vi "get-data.vi"(3 "error in (no error)":errorcluster, 4 "andor-get-data-cluster":T2={"detector"=0, "HBinning"=1, "readout mode"=0} {"readout mode" items=["Full Vertical Binning", "Image", "Vertical Binning"]; "HBinning" items=["1x"=1, "2x"=2, "4x"=4, "8x"=8, "16x"=16]; "detector" items=["Newton", "iDus", "Clara", "Xeva"]}, 5 "xeva-camref-in":T3) -> (0 "error out":errorcluster, 1 "raw-data":i32[](array[numeric]), 2 "xeva-camref-out":T3)   [LabVIEW 2015]
uses:
  <vilib>/Xenics Infrared Solutions/Xeneth LabVIEW API/VIs/Controls/Camara.ctl
  <userlib>/atmcd32d.llb/Error Code Enum typedef.ctl
  <vilib>/Xenics Infrared Solutions/Xeneth LabVIEW API/Xeneth.lvlib
panel:
  out "Get Data Status":T1=enum."DRV_SUCCESS"
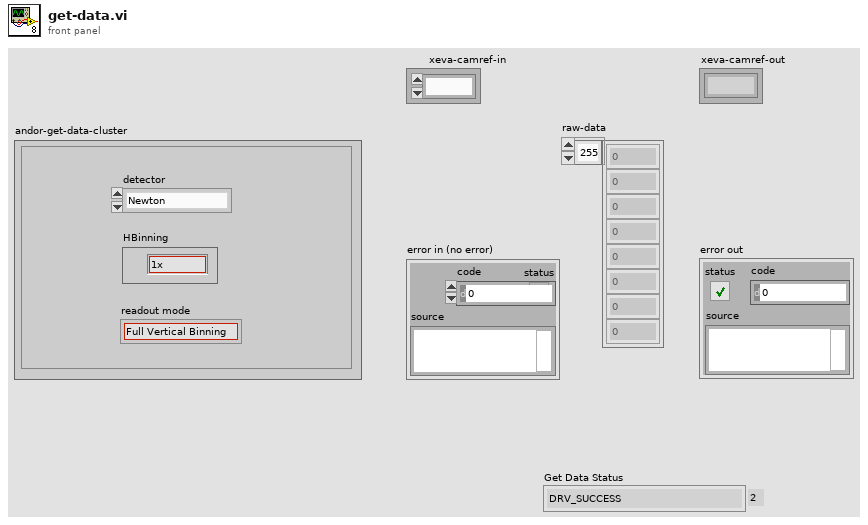
[diagram p1: front panel]
types:
  T1 = typedef "Error Code Enum typedef.ctl" = enum32{"N/A (0)", "DRV_ERROR_CODES", "DRV_SUCCESS", "DRV_VXDNOTINSTALLED", "DRV_ERROR_SCAN", "DRV_ERROR_CHECK_SUM", "DRV_ERROR_FILELOAD", "DRV_UNKNOWN_FUNC", "DRV_ERROR_VXD_INIT", "DRV_ERROR_ADDRESS", "DRV_ERROR_PAGELOCK", "DRV_ERROR_PAGEUNLOCK", "DRV_ERROR_BOARDTEST", "DRV_ERROR_ACK", "DRV_ERROR_UP_FIFO", "DRV_ERROR_PATTERN", "N/A (16)", "DRV_ACQUISITION_ERRORS", "DRV_ACQ_BUFFER", "DRV_ACQ_DOWNFIFO_FULL", "DRV_PROC_UNKONWN_INSTRUCTION", "DRV_ILLEGAL_OP_CODE", "DRV_KINETIC_TIME_NOT_MET", "DRV_ACCUM_TIME_NOT_MET", "DRV_NO_NEW_DATA", "N/A (25)", "DRV_SPOOLERROR", "N/A (27)", "N/A (28)", "N/A (29)", "N/A (30)", "N/A (31)", "N/A (32)", "DRV_TEMPERATURE_CODES", "DRV_TEMPERATURE_OFF", "DRV_TEMPERATURE_NOT_STABILIZED", "DRV_TEMPERATURE_STABILIZED", "DRV_TEMPERATURE_NOT_REACHED", "DRV_TEMPERATURE_OUT_RANGE", "DRV_TEMPERATURE_NOT_SUPPORTED", "DRV_TEMPERATURE_DRIFT", "N/A (41)", "N/A (42)", "N/A (43)", "N/A (44)", "N/A (45)", "N/A (46)", "N/A (47)", "N/A (48)", "DRV_GENERAL_ERRORS", "DRV_INVALID_AUX", "DRV_COF_NOTLOADED", "DRV_FPGAPROG", "DRV_FLEXERROR", "DRV_GPIBERROR", "N/A (55)", "N/A (56)", "N/A (57)", "N/A (58)", "N/A (59)", "N/A (60)", "N/A (61)", "N/A (62)", "N/A (63)", "DRV_DATATYPE", "DRV_DRIVER_ERRORS", "DRV_P1INVALID", "DRV_P2INVALID", "DRV_P3INVALID", "DRV_P4INVALID", "DRV_INIERROR", "DRV_COFERROR", "DRV_ACQUIRING", "DRV_IDLE", "DRV_TEMPCYCLE", "DRV_NOT_INITIALIZED", "DRV_P5INVALID", "DRV_P6INVALID", "DRV_INVALID_MODE", "DRV_INVALID_FILTER", "DRV_I2CERRORS", "DRV_I2CDEVNOTFOUND", "DRV_I2CTIMEOUT", "DRV_P7INVALID", "N/A (84)", "N/A (85)", "N/A (86)", "N/A (87)", "N/A (88)", "N/A (89)", "DRV_IOCERROR", "DRV_VRMVERSIONERROR"}
  T2 = cluster{"detector":u16, "HBinning":u16, "readout mode":u16}
  T3 = typedef "Xeneth.lvlib/Camara.ctl" = refnum<k1>
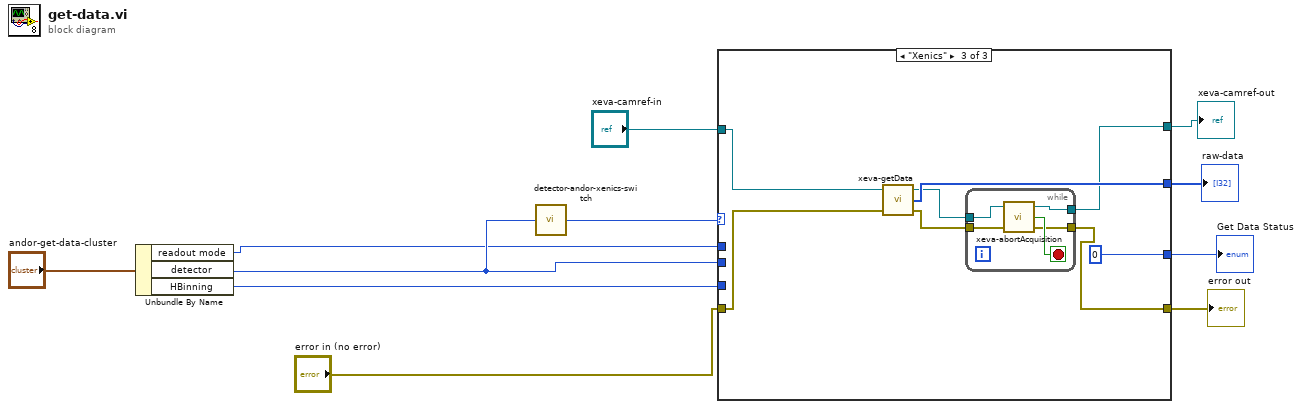
[diagram p0: block diagram]
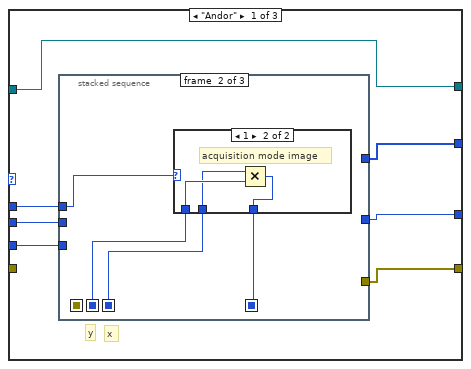
[diagram p2: hidden frame]
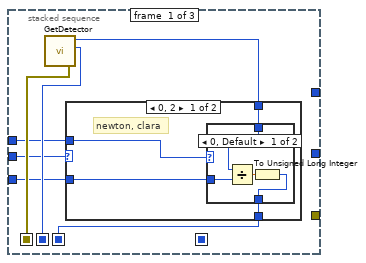
[diagram p3: hidden frame]
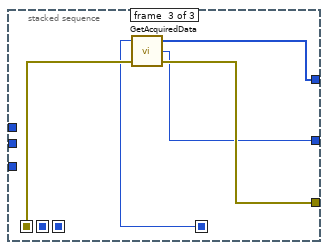
[diagram p7: hidden frame]
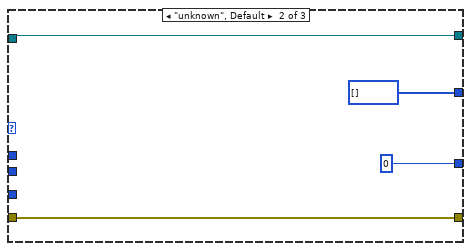
[diagram p8: hidden frame]
diagram:
  n1 = Unbundle By Name("andor-get-data-cluster") -> ("readout mode"=w5:u16, "detector"=w6:u16, "HBinning"=w4:u16)
  n2 = call "detector-andor-xenics-switch.vi"("Detector"=w6) -> ("Manufacturer"=w7:enum16{"Andor", "Xenics", "unknown"})
  n3 = case shown="\"Xenics\"" w7 {
    tunnel: [w13 w52 w53] -> w11
    tunnel: "error in (no error)" -> [_ w52 w59]
    tunnel: "xeva-camref-in" -> [w18 w51 w58]
    tunnel: [w18 w51 w55] -> w8
    tunnel: w5 -> [w17 _ _]
    tunnel: w4 -> [w16 _ _]
    tunnel: w6 -> [w15 _ _]
    tunnel: [w14 u32 0 ("DLL error code") u32 0 ("DLL error code")] -> w2
    tunnel: [w12 i32[] [] ("array") w57] -> w1
    frame "Andor" {
      # "x"
      # "y"
      n4 = stacked-sequence {
        seq-local: [w24 _ _] -> [_ w39 _]
        seq-local: [w23 _ _] -> [_ w38 _]
        seq-local: [_ w37 _] -> [_ _ w46]
        seq-local: [w22 _ _] -> [_ _ w48]
        tunnel: [_ _ w47] -> w13
        tunnel: [_ _ w45] -> w14
        tunnel: [_ _ w44] -> w12
        tunnel: w17 -> [w21 w36 _]
        tunnel: w16 -> [w20 _ _]
        tunnel: w15 -> [w19 _ _]
        frame #0 {
          n5 = call <userlib>:"GetDetector.vi"() -> ("error out"=w22:errorcluster, "ypixels"=w24:i32, "xpixels"=w25:i32)  [unwired: 4 in, 1 out]
          n6 = case shown="0, 2" w19 {
            tunnel: w25 -> [w29 w35]
            tunnel: [w28 w35] -> w23
            tunnel: w21 -> [w27 _]
            tunnel: w20 -> [w26 _]
            frame 0, 2 {
              # "newton, clara"
              n7 = case shown="0, Default" w27 {
                tunnel: w26 -> [w33 _]
                tunnel: w29 -> [w32 w34]
                tunnel: [w30 w34] -> w28
                frame 0, Default {
                  n8 = Divide(x=w32, y=w33) -> (x/y=w31:dbl)
                  n9 = To Unsigned Long Integer(number=w31) -> (unsigned 32bit integer=w30:u32)
                }
                frame 3 {
                  # "disabled\nfor image"
                }
              }
            }
            frame Default {
            }
          }
        }
        frame #1 {
          n10 = case shown="1" w36 {
            tunnel: w39 -> [_ w43]
            tunnel: w38 -> [w40 w42]
            tunnel: [w40 w41] -> w37
            frame 0, Default {
            }
            frame 1 {
              # "acquisition mode image"
              n11 = Multiply(x=w42, y=w43) -> (x*y=w41:u32)
            }
          }
        }
        frame #2 {
          n12 = call <userlib>:"GetAcquiredData.vi"("error in (no error)"=w48, "size"=w46) -> ("error out"=w47:errorcluster, "DLL error code"=w45:u32, "array"=w44:i32[])  [unwired: 1 in]
        }
      }
    }
    frame "unknown", Default {
    }
    frame "Xenics" {
      n13 = call "xeva-getData.vi"("error in (no error)"=w59, "xeva-camref-in"=w58) -> ("error out"=w54:errorcluster, "xeva-data"=w57:u16[], "xeva-camref-out"=w56:T3)  [unwired: 1 in]
      n14 = while {
        tunnel: w56 -> [w64]
        tunnel: [w63] -> w55
        tunnel: w54 -> [w62]
        tunnel: [w61] -> w53
        stop <- w65 stop-if-true
        n15 = call "xeva-abortAcquisition.vi"("error in (no error)"=w62, "Cam Ref"=w64) -> ("error out"=w61:errorcluster, "aborted"=w65:bool, "Cam Ref Out"=w63:T3)  [unwired: 1 in]
      }
    }
  }
  "error out" <- w11
  "xeva-camref-out" <- w8
  "Get Data Status" <- w2
  "raw-data" <- w1
